vi "FrequencyCounter Example.vi"() -> ()   [LabVIEW 2012, in "Phidget Frequency Counter.lvlib"]
uses:
  <instrlib>/Phidgets/Phidget Frequency Counter/Phidget Frequency Counter.lvlib
  <instrlib>/Phidgets/Phidget Frequency Counter/Public/FrequencyCounterStart.vi
  <instrlib>/Phidgets/Phidget Frequency Counter/Public/FrequencyCounterClose.vi
  <instrlib>/Phidgets/Phidget Common/Phidget Common.lvlib
panel:
  out "Frequency":dbl
  in  "stop":bool
  out "Time Elapsed":dbl
  out "Count":i64
  out "error out":errorcluster
  in  "error in (no error)":errorcluster
  in  "Device Info":T1={"Serial Number"=-1, "Channel"=0, "Port"=0}
  out "Attached?":bool
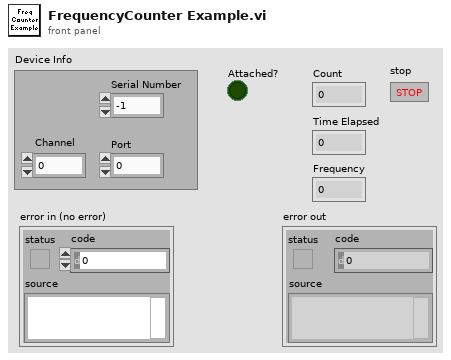
[diagram p1: front panel]
types:
  T1 = cluster{"Serial Number":i32, "Channel":i32, "Port":i32}
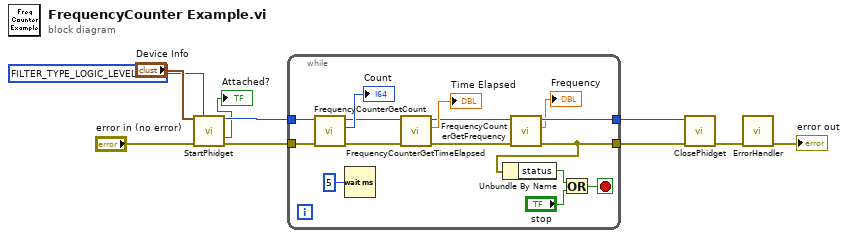
[diagram p0: block diagram]
diagram:
  w1 = u32 2 items=["FILTER_TYPE_ZERO_CROSSING"=1, "FILTER_TYPE_LOGIC_LEVEL"=2] ("Filter Type")
  n1 = call-poly <instrlib>:"StartPhidget.vi"("Device Info"="Device Info", "Filter Type"=w1, "error in (no error)"="error in (no error)") -> ("Phidget ID"=w4:u64, "Attached?"=→"Attached?":bool, "error out"=w3:errorcluster)  [unwired: 9 in, 1 out]
  n2 = while {
    tunnel: [w16] -> w6
    tunnel: [w11] -> w5
    tunnel: w4 -> [w24]
    tunnel: w3 -> [w23]
    stop <- w12 stop-if-true
    n3 = call <instrlib>:"FrequencyCounterGetCount.vi"("error in (no error)"=w23, "Device In"=w24) -> ("error out"=w21:errorcluster, "Count"=→"Count":i64, "Device Out"=w22:u64)  [unwired: 6 in]
    n4 = Wait (ms)(milliseconds to wait=u32 5) -> ()  [unwired: 1 out]
    n5 = call <instrlib>:"FrequencyCounterGetTimeElapsed.vi"("error in (no error)"=w21, "Device In"=w22) -> ("error out"=w17:errorcluster, "Time Elapsed"=→"Time Elapsed":dbl, "Device Out"=w18:u64)  [unwired: 6 in]
    n6 = call <instrlib>:"FrequencyCounterGetFrequency.vi"("error in (no error)"=w17, "Device In"=w18) -> ("error out"=w11:errorcluster, "Frequency"=→"Frequency":dbl, "Device Out"=w16:u64)  [unwired: 6 in]
    n7 = Unbundle By Name(w11) -> ("status"=w14:bool)
    n8 = Or(x=w14, y="stop") -> (x .or. y?=w12:bool)
  }
  n9 = call-poly <instrlib>:"ClosePhidget.vi"("error in"=w5, "Device In"=w6) -> ("error out"=w8:errorcluster)  [unwired: 9 in]
  n10 = call <instrlib>:"ErrorHandler.vi"("error in"=w8) -> ("error out"=→"error out":errorcluster)  [unwired: 9 in, 1 out]
